vi "AnalyseTVE.vi"(1 "NISTPhasor":T1, 2 "FlukePhasor":T1) -> (6 "TVE":dbl)   [LabVIEW 2014]
uses:
  typedefs/PhasorRectangular.ctl
  <vilib>/Analysis/NI_AAL_Angle.lvlib
  <vilib>/Analysis/coordinate.llb/Wrap Angle (scalar).vi
  <vilib>/Analysis/coordinate.llb/Angle Units.ctl
  <vilib>/Analysis/coordinate.llb/Angle Range (Degree).ctl
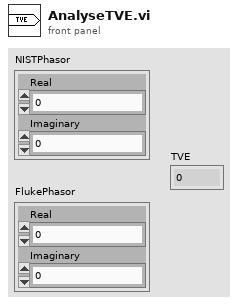
[diagram p1: front panel]
types:
  T1 = typedef "PhasorRectangular.ctl" = cluster{"Real":dbl, "Imaginary":dbl}
  T2 = typedef "NI_AAL_Angle.lvlib/Angle Range (Degree).ctl" = u16
  T3 = typedef "NI_AAL_Angle.lvlib/Angle Units.ctl" = i32
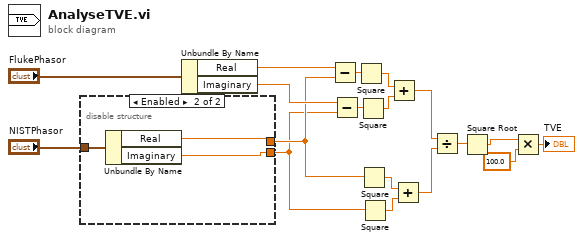
[diagram p0: block diagram]
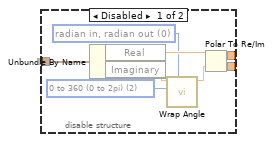
[diagram p2: hidden frame]
diagram:
  n1 = disable-structure shown="Enabled" {
    disable-tunnel: "NISTPhasor" -> [w26 w29]
    disable-tunnel: [w24 w28] -> w4
    disable-tunnel: [w23 w27] -> w3
    frame Disabled {
      w19 = T2 2 items=["none", "-180 to 180 (-pi to pi)", "0 to 360 (0 to 2pi)"] ("angle range")
      w20 = T3 0 items=["radian in, radian out", "radian in, degree out", "degree in, degree out", "degree in, radian out"] ("angle units")
      n2 = Unbundle By Name(w26) -> ("Real"=w25:dbl, "Imaginary"=w22:dbl)
      n3 = call-poly <vilib>:"Wrap Angle.vi"("angle units"=w20, "angle range"=w19, "angle in"=w22) -> ("angle out"=w21:dbl)  [unwired: 7 in, 1 out]
      n4 = Polar To Re/Im(2:w21, 3:w25) -> (0:w23:dbl, 1:w24:dbl)
    }
    frame Enabled {
      n5 = Unbundle By Name(w29) -> ("Real"=w28:dbl, "Imaginary"=w27:dbl)
    }
  }
  n6 = Unbundle By Name("FlukePhasor") -> ("Real"=w6:dbl, "Imaginary"=w5:dbl)
  n7 = Subtract(x=w6, y=w4) -> (x-y=w16:dbl)
  n8 = Subtract(x=w5, y=w3) -> (x-y=w15:dbl)
  n9 = Square(x=w16) -> (x^2=w14:dbl)
  n10 = Square(x=w15) -> (x^2=w13:dbl)
  n11 = Square(x=w4) -> (x^2=w11:dbl)
  n12 = Square(x=w3) -> (x^2=w12:dbl)
  n13 = Add(x=w14, y=w13) -> (x+y=w9:dbl)
  n14 = Add(x=w11, y=w12) -> (x+y=w10:dbl)
  n15 = Divide(x=w9, y=w10) -> (x/y=w8:dbl)
  n16 = Square Root(x=w8) -> (sqrt(x)=w7:dbl)
  n17 = Multiply(x=w7, y=100.0) -> (x*y=→"TVE":dbl)
